vi "Stop Chassis.vi"(8 "error in (no error)":errorcluster, 10 "final error code":i32, 11 "LS Only in":refnum<class "LS Only.lvclass">) -> (0 "error out":errorcluster, 2 "Max Read Time (ms)":i32, 3 "LS Only out":refnum<class "LS Only.lvclass">)   [LabVIEW 2012, in "Data Acquisition.lvlib" / "LS Only.lvclass"]
uses:
  LS Only.lvclass
  Class Chassis Tasks/Chassis Tasks.lvclass/Chassis Tasks.ctl
  <vilib>/ActorFramework/Stop Msg/Stop Msg.lvclass/Stop Msg.ctl
  <vilib>/ActorFramework/Message Enqueuer/Message Enqueuer.lvclass/Message Enqueuer.ctl
  Class Chassis Tasks/Read LS DAQ Task.vi
  Class Chassis Tasks/Read LS ActorQ.vi
  <vilib>/ActorFramework/Stop Msg/Send Emergency Stop.vi
  <vilib>/ActorFramework/Stop Msg/Send Normal Stop.vi
  <vilib>/ActorFramework/Message Enqueuer/Enqueue Critical.vi
  <vilib>/ActorFramework/Message Enqueuer/Enqueue.vi
  <vilib>/ActorFramework/Message Priority Queue/Priority Enqueue.vi
  <vilib>/ActorFramework/Message Enqueuer/Message Enqueuer.lvclass
  <vilib>/ActorFramework/Stop Msg/Stop Msg.lvclass
  Class DAQ Task/DAQ Task.lvclass
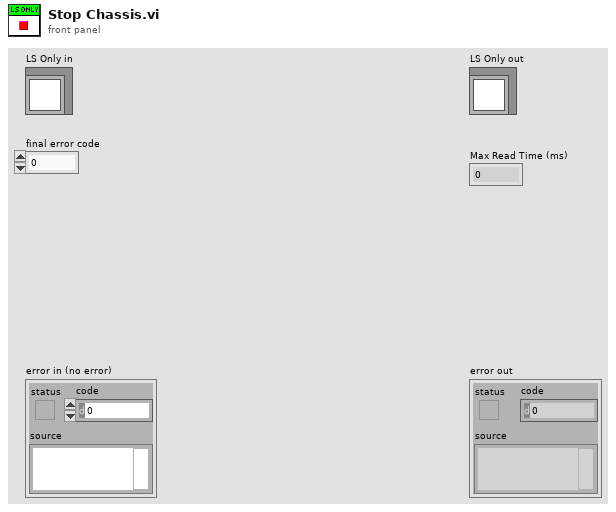
[diagram p1: front panel]
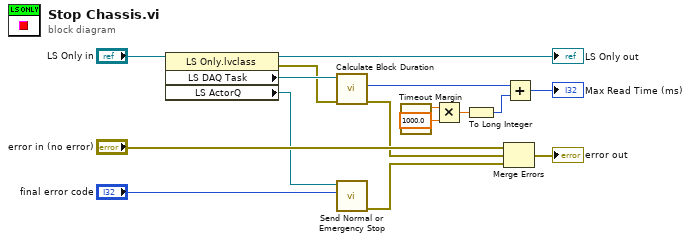
[diagram p0: block diagram]
diagram:
  n1 = property class="LS Only.lvclass"(reference="LS Only in") -> (reference out=→"LS Only out":refnum<class "LS Only.lvclass">, error out=w8:errorcluster, "LS DAQ Task"=w9:refnum<class "DAQ Task.lvclass">, "LS ActorQ"=w10:refnum<class "Message Enqueuer.lvclass">)  [unwired: 1 in]
  n2 = call "Calculate Block Duration.vi"("error in (no error)"=w8, "DAQ Task in"=w9) -> ("error out"=w7:errorcluster, "Block Duration (ms)"=w3:i32)  [unwired: 7 in, 1 out]
  n3 = call <vilib>:"Send Normal or Emergency Stop.vi"("final error code"="final error code", "Message Enqueuer"=w10) -> ("error out"=w16:errorcluster)  [unwired: 9 in]
  n4 = call "Timeout Margin.vi"() -> ("y"=w6:dbl)  [unwired: 11 in]
  n5 = Multiply(x=w6, y=1000.0) -> (x*y=w4:dbl)
  n6 = To Long Integer(number=w4) -> (32bit integer=w2:i32)
  n7 = Merge Errors("error in (no error)", w7, w16) -> (→"error out":errorcluster)
  n8 = Add(x=w3, y=w2) -> (x+y=→"Max Read Time (ms)":i32)
